vi "Thermo Channel UI.vi"() -> ()   [LabVIEW 2025, in "Thermo.lvlib" / "Thermo Channel.lvclass"]
doc: "Copyright 2017 National Instruments Corporation\n\nLicensed under the Apache License, Version 2.0 (the \"License\"); you may not use this file except in compliance with the License. You may obtain a copy of the License at http://www.apache.org/licenses/LICENSE-2.0\nUnless required by applicable law or agreed to in writing, software distributed under the License is distributed on an \"AS IS\" BASIS, WITHOUT WARRANTIES OR CONDITIONS OF ANY KIND, either express or implied. See the License for the specific language governing permissions and limitations under the License."
uses:
  Thermo Channel.lvclass
  Thermo Channel.lvclass/Thermo Channel.ctl
  C:/Users/Public/Documents/Sandia National Labs/TSS Plugin/Abstract Engine.lvlibp/Plugin/Abstract/Abstract Channel/Abstract Channel.lvclass
  C:/Users/Public/Documents/Sandia National Labs/TSS Plugin/CEF.lvlibp/serializable node/CEF_serializable node.lvclass
  C:/Users/Public/Documents/Sandia National Labs/TSS Plugin/CEF.lvlibp/Node/CEF_Node.lvclass
  C:/Working copy/tss/Plugin/Engines/Thermo/Thermo Channel/Thermo Channel.lvclass
  Users/Public/Documents/Sandia National Labs/TSS Plugin/CEF.lvlibp/Node/CEF_Node.lvclass
  Thermo Channel configuration/Thermo Channel configuration.lvclass
  Users/Public/Documents/Sandia National Labs/TSS Plugin/CEF.lvlibp/Node/NodeRef.ctl
  Users/Public/Documents/Sandia National Labs/TSS Plugin/CEF.lvlibp/Node/UserEventRef.ctl
  Users/Public/Documents/Sandia National Labs/TSS Plugin/CEF.lvlibp/Node/mainQref.ctl
  Thermo Channel configuration/Channel Setting.ctl
  Users/Public/Documents/Sandia National Labs/TSS Plugin/Abstract Engine.lvlibp/Plugin/Abstract/Channel configuration/Default Channel.ctl
  Users/Public/Documents/Sandia National Labs/TSS Plugin/Abstract Engine.lvlibp/Plugin/Abstract/Channel configuration/Channel configuration.lvclass
panel:
  in  "Thermo Channel":cluster{"Default":T1, "Setting":T2}={"Default"={"Address"="None", "SW Alias"="None", "Enabled"=TRUE, "Type"="None", "Description"="* Type = Channel Class"}, "Setting"={"Numeric"=0.5, "Combo"="", "String"="", "Boolean"=FALSE}} {"Setting"."Numeric" format="%#_f"}
  in  "user event":T3
  in  "main queue":T4
  in  "node ref":T5
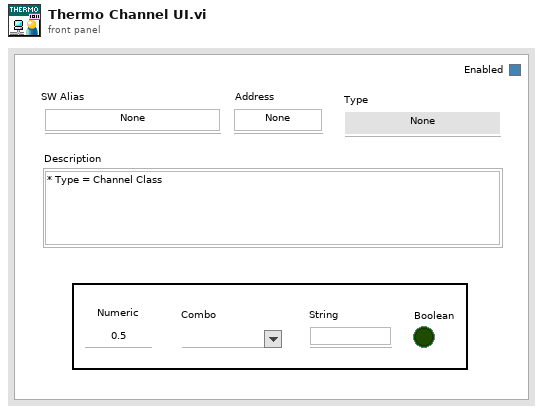
[diagram p1: front panel]
types:
  T1 = typedef "Abstract Engine.lvlibp/Channel configuration.lvclass/Default Channel.ctl" = cluster{"Address":string, "SW Alias":string, "Enabled":bool, "Type":string, "Description":string}
  T2 = typedef "Thermo.lvlib/Thermo Channel configuration.lvclass/Channel Setting.ctl" = cluster{"Numeric":dbl, "Combo":string, "String":string, "Boolean":bool}
  T3 = typedef "CEF.lvlibp/CEF_Node.lvclass/UserEventRef.ctl" = refnum<user-event>
  T4 = typedef "CEF.lvlibp/CEF_Node.lvclass/mainQref.ctl" = refnum<queue>
  T5 = typedef "CEF.lvlibp/CEF_Node.lvclass/NodeRef.ctl" = refnum<data-value>
  T6 = cluster{"Channel Setting":T1, "Thermo Channel Setting":T2}
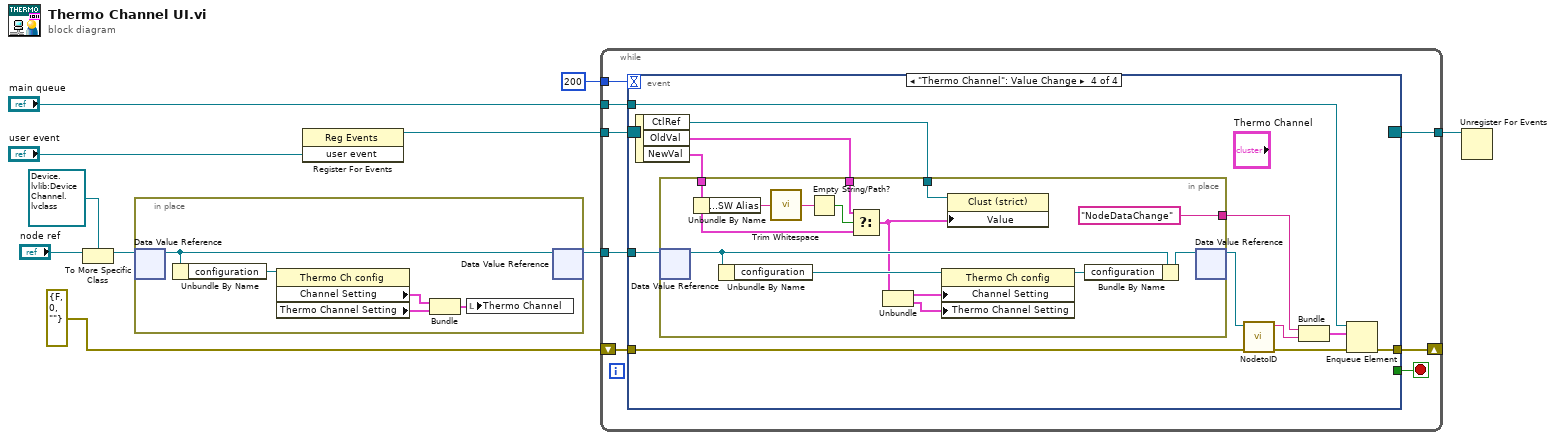
[diagram p0: block diagram]
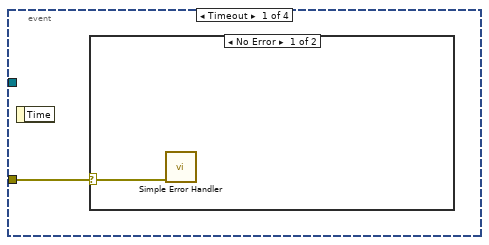
[diagram p2: hidden frame]
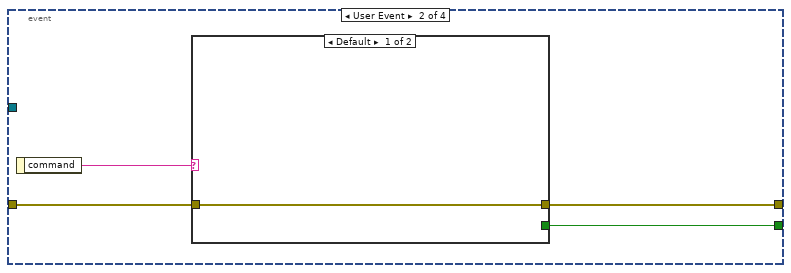
[diagram p4: hidden frame]
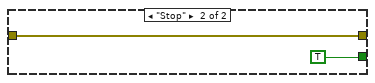
[diagram p5: hidden frame]
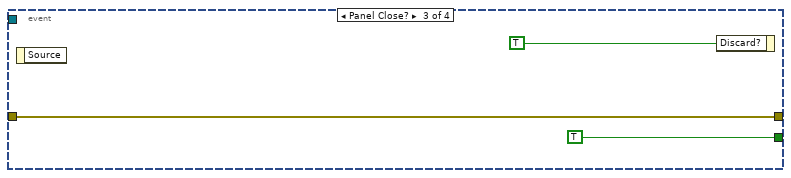
[diagram p6: hidden frame]
diagram:
  n1 = To More Specific Class(target class=refnum<data-value> refnum ("data value reference"), reference="node ref") -> (specific class reference=w6:refnum<data-value>)  [unwired: 1 in, 1 out]
  n2 = in-place {
    # "Initialize the front panel controls when loaded"
    n3 = in-place-dvr #1(w6) -> (w15:refnum<class "Thermo Channel.lvclass">)  [unwired: 1 out]
    n4 = Unbundle By Name(w15) -> ("configuration"=w14:refnum<class "Thermo Channel configuration.lvclass">)
    n5 = property class="Thermo Ch config"(reference=w14) -> ("Channel Setting"=w13:T1, "Thermo Channel Setting"=w12:T2)  [unwired: 1 in, 2 out]
    n6 = Bundle("Channel Setting"=w13, "Thermo Channel Setting"=w12) -> (w11:T6)  [unwired: 1 in]
    n7 = local write "Thermo Channel"(w11) -> ()
    n8 = in-place-dvr #1(w15) -> (w5:refnum<data-value>)  [unwired: 1 out]
  }
  n9 = register-events("user event") -> (reference out=w9:refnum<event-registration>)  [unwired: 2 in, 1 out]
  n10 = while {
    tunnel: w5 -> [w23]
    tunnel: w9 -> [w22]
    tunnel: [w21] -> w8
    tunnel: "main queue" -> [w17]
    shift-right: [w18] -> _
    shift-left: errorcluster {"status"=FALSE, "code"=0, "source"=""} ("error out") -> [w19]
    tunnel: 200 -> [w16]
    stop <- w20 stop-if-true
    n11 = event shown="[3] \"Thermo Channel\": Value Change" {
      selector: w22 -> [_ _ _ _]
      dyn-events: [_ _ _ _] -> w21
      timeout: w16 -> [_ _ _ _]
      tunnel: w23 -> [_ _ _ w44]
      tunnel: [_ w29 TRUE _] -> w20
      tunnel: [_ w26 w33 w42] -> w18
      tunnel: w19 -> [w24 w28 w33 w37]
      tunnel: w17 -> [_ _ _ w41]
      event Timeout {
        n12 = event-data() -> ()  [unwired: 1 in, 1 out]
        n13 = case shown="No Error" w24 {
          selector: w24 -> [w25 _]
          frame No Error {
            n14 = call <vilib>:"Simple Error Handler.vi"("error in (no error)"=w25) -> ()  [unwired: 4 in, 5 out]
          }
          frame Error {
          }
        }
      }
      event User Event {
        n15 = event-data() -> ("command"=w27:string)  [unwired: 1 in]
        n16 = case shown="Default" w27 {
          tunnel: [_ TRUE] -> w29
          tunnel: w28 -> [w30 w31]
          tunnel: [w30 w31] -> w26
          frame Default {
          }
          frame "Stop" {
          }
        }
      }
      event Panel Close? {
        n17 = event-data() -> ()  [unwired: 1 in, 1 out]
        n18 = event-data("Discard?"=TRUE) -> ()  [unwired: 1 in, 1 out]
      }
      event "Thermo Channel": Value Change {
        n19 = event-data() -> ("CtlRef"=w45:refnum<vi>, "OldVal"=w46:cluster{"Default":T1, "Setting":T2}, "NewVal"=w47:cluster{"Default":T1, "Setting":T2})  [unwired: 1 in]
        n20 = in-place {
          in-place-border: w46 -> [w57]
          in-place-border: w47 -> [w54]
          in-place-border: w45 -> [w56]
          in-place-border: ["NodeDataChange" ("Message Name")] -> w40
          n21 = in-place-dvr #2(w44) -> (w61:refnum<class "Thermo Channel.lvclass">)  [unwired: 1 out]
          n22 = Unbundle By Name(w54) -> ("Default.SW Alias"=w55:string)
          n23 = Unbundle By Name(w61) -> ("configuration"=w59:refnum<class "Thermo Channel configuration.lvclass">)
          n24 = call <vilib>:"Trim Whitespace.vi"("string"=w55) -> ("trimmed string"=w52:string)  [unwired: 1 in]
          n25 = Empty String/Path?(string/path=w52) -> (empty?=w53:bool)
          n26 = Select(t=w57, s=w53, f=w54) -> (s? t:f=w51:cluster{"Default":T1, "Setting":T2})
          n27 = Unbundle(w51) -> ("Default"=w48:T1, "Setting"=w50:T2)
          n28 = property class="Thermo Ch config"(reference=w59, "Channel Setting"=w48, "Thermo Channel Setting"=w50) -> (reference out=w58:refnum<class "Thermo Channel configuration.lvclass">)  [unwired: 1 in, 1 out]
          n29 = property class="Clust (strict)"(reference=w56, "Value"=w51) -> ()  [unwired: 1 in, 2 out]
          n30 = Bundle By Name(cluster=w61, "configuration"=w58) -> (w60:refnum<class "Thermo Channel.lvclass">)
          n31 = in-place-dvr #2(w60) -> (w43:refnum<data-value>)  [unwired: 1 out]
        }
        n32 = call "NodetoID.vi"("error in"=w37, "node ref"=w43) -> ("error out"=w36:errorcluster, "ID"=w39:string)  [unwired: 8 in]
        n33 = Bundle("Message Name"=w40, "ID"=w39) -> (w38:cluster{"Message Name":string, "ID":string})  [unwired: 1 in]
        n34 = Enqueue Element(queue=w41, element=w38, error in (no error)=w36) -> (error out=w42:errorcluster)  [unwired: 1 in, 2 out]
      }
    }
  }
  n35 = Unregister For Events(event registration refnum=w8) -> ()  [unwired: 1 in, 1 out]
